vi "PrefDialog.vi"(8 "error in (no error)":errorcluster, 11 "SpecAnPlugins.lvlib":refnum<class "SpecAnBase.lvclass">) -> (0 "error out":errorcluster, 2 "Change Occured?":bool, 3 "SpecAnPlugins.lvlib":refnum<class "SpecAnBase.lvclass">)   [LabVIEW 2018, in "SpecAnPlugins.lvlib" / "SpecAnBase.lvclass"]
doc: "This VI opens up the modal preference dialog window and allows a user to configure the dialog based on a new configuration or the existing configuration that was loaded"
uses:
  SpecAnBase.lvclass
  C:/Program Files (x86)/National Instruments/LabVIEW 2018/user.lib/NIST/BaseClasses/BasePlugin_class/BasePlugin.lvclass
  <userlib>/NIST/BaseClasses/BasePlugin_class/BasePlugin.lvclass/BasePlugin.ctl
  <userlib>/NIST/BaseClasses/BasePlugin_class/Accessors/Read PluginIniFilePath.vi
  <userlib>/NIST/BaseClasses/BasePlugin_class/Accessors/Write PluginIniFilePath.vi
  <vilib>/Utility/config.llb/NI_LVConfig.lvlib
panel:
  in  "btnSave As":bool
  in  "btnSave":bool
  in  "Tab Control":T1(tab)
  in  "Acquisition":T2
  in  "Frequency":T3
  in  "Level":T4
  in  "SweepCoupling":T5
  in  "Trace":T6(array[cluster])
  in  "Trigger":T7
  in  "btnCancel":bool
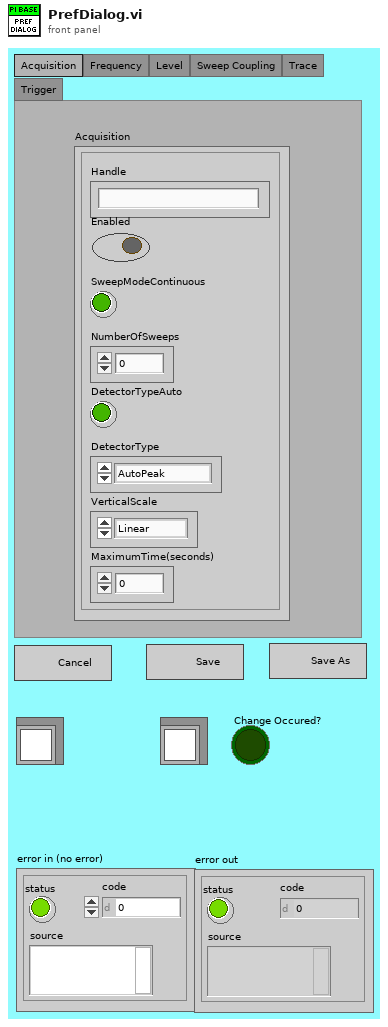
[diagram p1: front panel]
types:
  T1 = enum32{"Acquisition", "Frequency", "Level", "Sweep Coupling", "Trace", "Trigger"}
  T2 = cluster{"Handle":string, "Connected":bool, "Enabled":bool, "SweepModeContinuous":bool, "NumberOfSweeps":i32, "DetectorTypeAuto":bool, "DetectorType":enum16{"AutoPeak", "Average", "MaximumPeak", "MinimumPeak", "Sample", "RMS"}, "VerticalScale":enum16{"Linear", "Logarithmic"}, "MaximumTime(seconds)":dbl}
  T3 = cluster{"FrequencyStart":dbl, "FrequencyStop":dbl, "FrequencyOffset":dbl}
  T4 = cluster{"InputImpedance":dbl, "AttenuationAuto":bool, "AmplitudeUnits":enum16{"dBm", "dBmV", "dBuV", "Volt", "Watt"}, "ReferenceLevel":dbl, "Attenuation":dbl, "ReferenceLevelOffset":dbl}
  T5 = cluster{"ResolutionBandwidth":dbl, "ResolutionBandwidthAuto":bool, "SweepTime":dbl, "VideoBandwidth":dbl, "VideoBandwidthAuto":bool, "SweepTimeAuto":bool}
  T6 = cluster{"TraceName":string, "TraceSize":i32, "TraceType":enum16{"Clear Write", "Maximum Hold", "Minimum Hold", "Video Average", "View", "Store"}}[]
  T7 = cluster{"TriggerSource":string, "TriggerLevel":dbl, "TriggerSlope":enum16{"Positive", "Negative"}}
  T8 = enum8{"Enabled", "Disabled", "Disabled and Grayed Out"}
  T9 = enum32{"Invalid", "Default", "Floating", "Floating/Auto-Hide", "Modal"}
  T10 = typedef "NI_LVConfig.lvlib/Config Data RefNum.ctl" = refnum<k1>
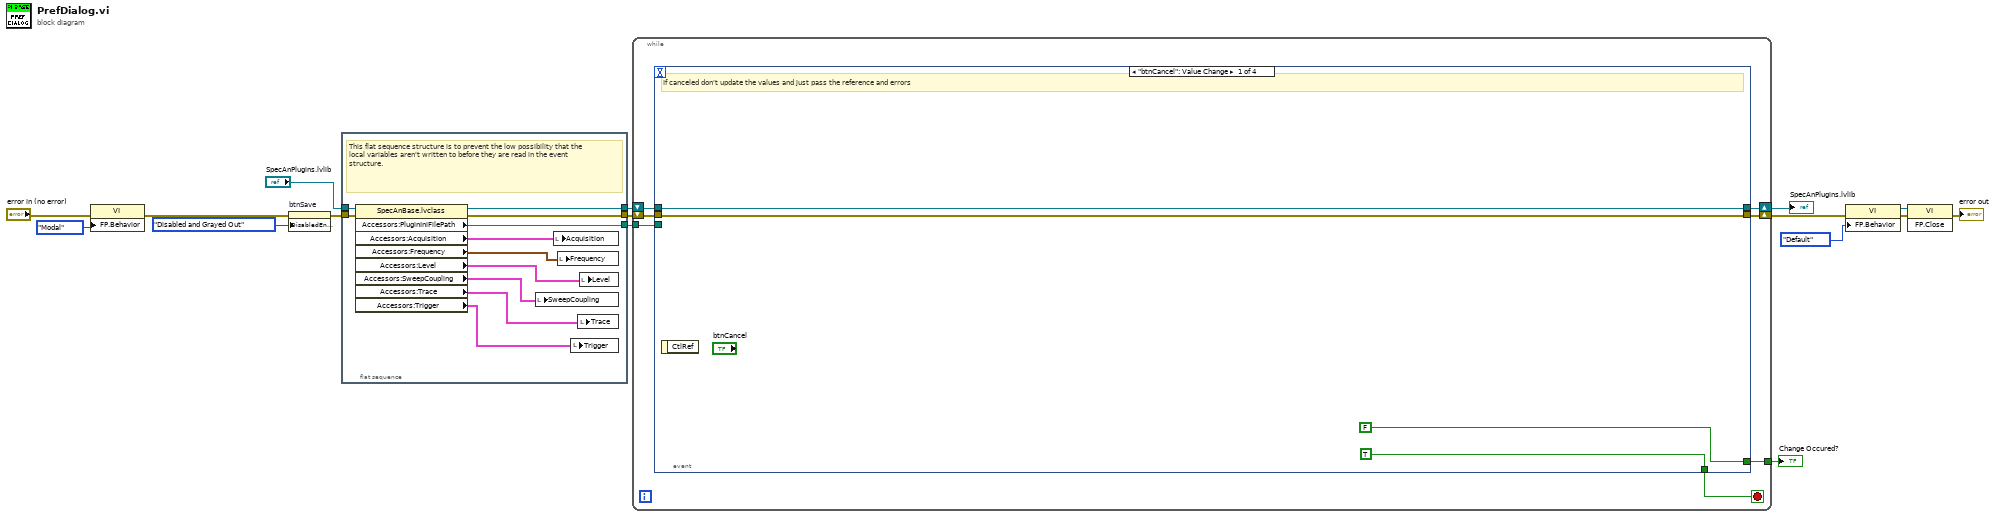
[diagram p0: block diagram]
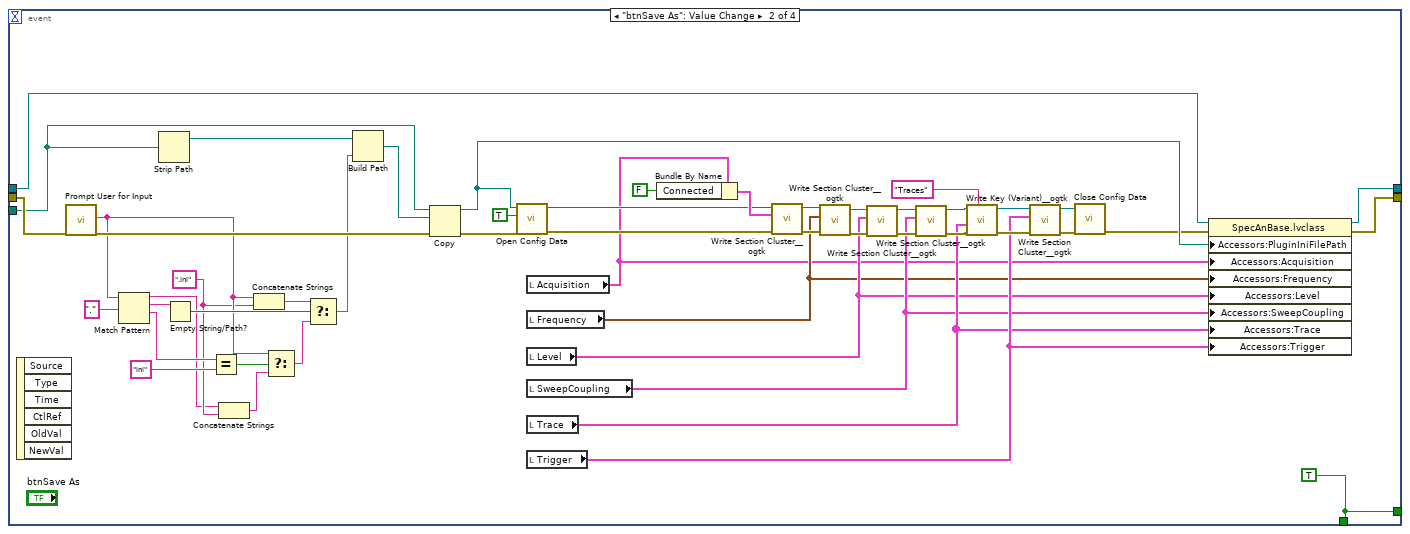
[diagram p2: hidden frame]
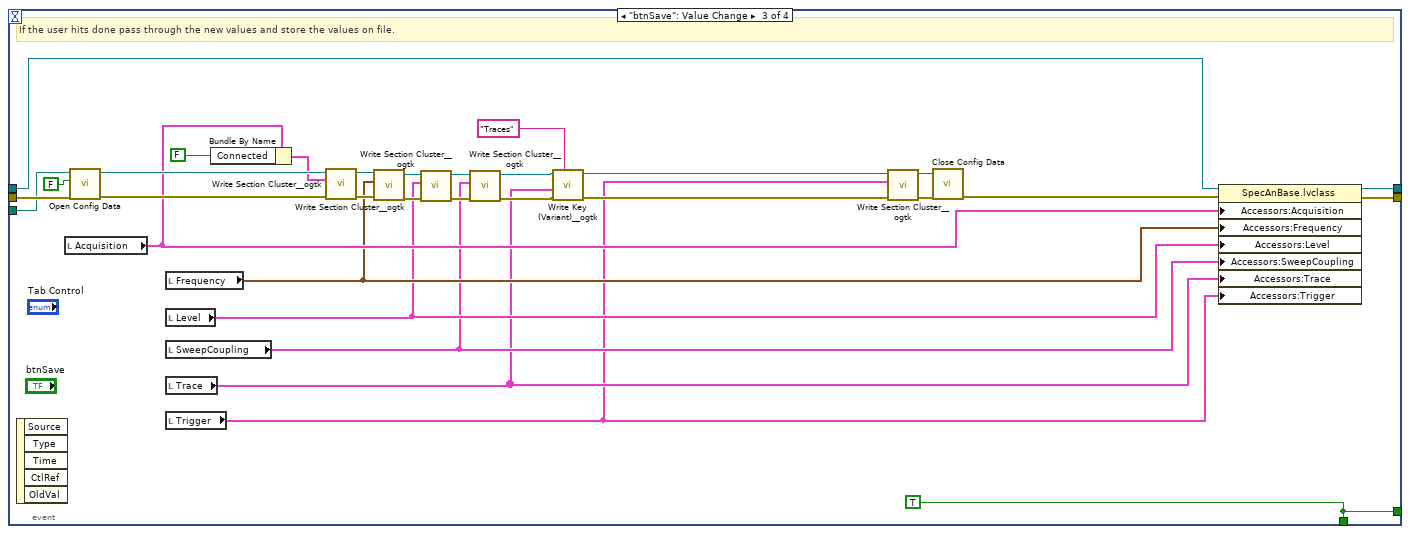
[diagram p3: hidden frame]
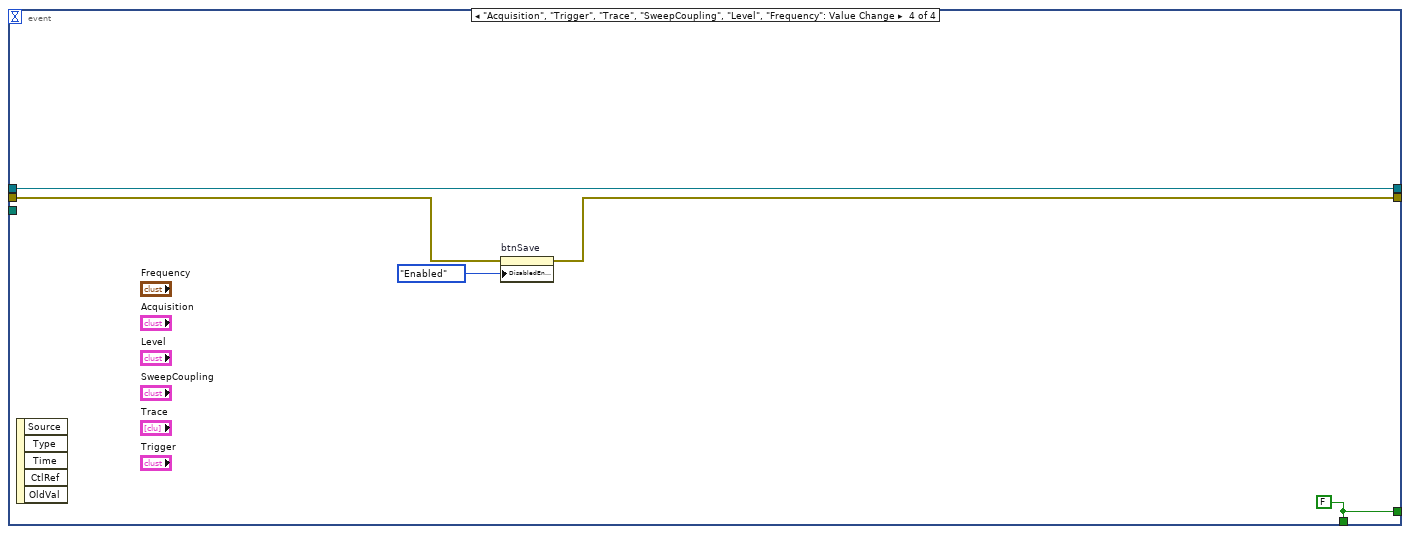
[diagram p4: hidden frame]
diagram:
  n1 = property class="VI"(error in="error in (no error)", "FP.Behavior"=T9."Modal" ("Front Panel Window:Behavior")) -> (error out=w1:errorcluster)  [unwired: 1 in, 1 out]
  n2 = property on="btnSave" class="Bool"(error in=w1, "DisabledEnum"=T8."Disabled and Grayed Out" ("Disabled")) -> (error out=w3:errorcluster)  [unwired: 1 in, 1 out]
  n3 = flat-sequence {
    tunnel: "SpecAnPlugins.lvlib" -> [w27]
    tunnel: w3 -> [w26]
    tunnel: [w25] -> w9
    tunnel: [w24] -> w8
    tunnel: [w23] -> w7
    frame #0 {
      # "This flat sequence structure is to prevent the low possibility that the local variables aren't written to before they are read in the event structure."
      n4 = property class="SpecAnBase.lvclass"(reference=w27, error in=w26) -> (reference out=w24:refnum<class "SpecAnBase.lvclass">, error out=w25:errorcluster, "Accessors:PluginIniFilePath"=w23:path, "Accessors:Acquisition"=w22:T2, "Accessors:Frequency"=w21:T3, "Accessors:Level"=w20:T4, "Accessors:SweepCoupling"=w19:T5, "Accessors:Trace"=w18:T6, "Accessors:Trigger"=w17:T7)
      n5 = local write "SweepCoupling"(w19) -> ()
      n6 = local write "Acquisition"(w22) -> ()
      n7 = local write "Frequency"(w21) -> ()
      n8 = local write "Trigger"(w17) -> ()
      n9 = local write "Trace"(w18) -> ()
      n10 = local write "Level"(w20) -> ()
    }
  }
  n11 = while {
    tunnel: w7 -> [w32]
    shift-right: [w30] -> w5
    shift-left: w9 -> [w34]
    shift-right: [w31] -> w6
    shift-left: w8 -> [w33]
    tunnel: [w28] -> w4
    stop <- w29 stop-if-true
    n12 = event shown="[0] \"btnCancel\": Value Change" {
      selector: _ -> [_ _ _ _]
      dyn-events: _ -> [_ _ _ _]
      timeout: _ -> [_ _ _ _]
      tunnel: w34 -> [w37 w84 w110 w122]
      tunnel: w33 -> [w38 w47 w118 w123]
      tunnel: w32 -> [_ w82 w102 _]
      tunnel: [w38 w86 w117 w123] -> w31
      tunnel: [w37 w85 w116 w121] -> w30
      tunnel: [TRUE w87 w94 w119] -> w29
      tunnel: [FALSE w87 w94 w119] -> w28
      event "btnCancel": Value Change {
        # "If canceled don't update the values and just pass the reference and errors"
        n13 = event-data() -> ()  [unwired: 1 in, 1 out]
      }
      event "btnSave As": Value Change {
        w69 = ".ini" ("string")
        w87 = TRUE
        n14 = event-data() -> ()  [unwired: 1 in, 6 out]
        n15 = call "Prompt User for Input"("error in (no error)"=w84) -> ("File Name"=w75:string, "error out"=w80:errorcluster)  [unwired: 15 in, 2 out]
        n16 = Match Pattern(string=w75, regular expression="." ("string")) -> (before substring=w68:string, match substring=w72:string, after substring=w71:string)  [unwired: 1 in, 1 out]
        n17 = Strip Path(path=w82) -> (stripped path=w83:path)  [unwired: 1 out]
        n18 = Empty String/Path?(string/path=w72) -> (empty?=w79:bool)
        n19 = Equal?(x=w71, y="ini" ("string")) -> (x = y?=w76:bool)
        n20 = Concatenate Strings(w68, w69) -> (w67:string)
        n21 = Concatenate Strings(w75, w69) -> (w78:string)
        n22 = Select(t=w75, s=w76, f=w67) -> (s? t:f=w74:string)
        n23 = Select(t=w78, s=w79, f=w74) -> (s? t:f=w77:string)
        n24 = Build Path(base path=w83, name or relative path=w77) -> (appended path=w81:path)
        n25 = Copy(8:w80, 10:w81, 11:w82) -> (0:w65:errorcluster, 3:w64:path)  [unwired: 2 in, 1 out]
        n26 = call <vilib>:"Open Config Data.vi"("error in (no error)"=w65, "create file if necessary (T)"=TRUE, "configuration file path"=w64) -> ("error out"=w46:errorcluster, "refnum"=w45:T10)  [unwired: 6 in, 1 out]
        n27 = local read "Acquisition"() -> (w39:T2)
        n28 = local read "Frequency"() -> (w40:T3)
        n29 = local read "Level"() -> (w41:T4)
        n30 = local read "SweepCoupling"() -> (w42:T5)
        n31 = local read "Trace"() -> (w43:T6)
        n32 = local read "Trigger"() -> (w44:T7)
        n33 = Bundle By Name(cluster=w39, "Connected"=FALSE) -> (w51:T2)
        n34 = call <userlib>:"Write Section Cluster__ogtk.vi"("error in (no error)"=w46, "Section Formatted Cluster"=w51, "refnum"=w45) -> ("error out"=w63:errorcluster, "dup refnum"=w62:T10)  [unwired: 7 in]
        n35 = call <userlib>:"Write Section Cluster__ogtk.vi"("error in (no error)"=w63, "Section Formatted Cluster"=w40, "refnum"=w62) -> ("error out"=w61:errorcluster, "dup refnum"=w60:T10)  [unwired: 7 in]
        n36 = call <userlib>:"Write Section Cluster__ogtk.vi"("error in (no error)"=w61, "Section Formatted Cluster"=w41, "refnum"=w60) -> ("error out"=w59:errorcluster, "dup refnum"=w58:T10)  [unwired: 7 in]
        n37 = call <userlib>:"Write Section Cluster__ogtk.vi"("error in (no error)"=w59, "Section Formatted Cluster"=w42, "refnum"=w58) -> ("error out"=w55:errorcluster, "dup refnum"=w54:T10)  [unwired: 7 in]
        n38 = call <userlib>:"Write Key (Variant)__ogtk.vi"("section"="Traces", "error in (no error)"=w55, "key-value"=w43, "refnum"=w54) -> ("error out"=w53:errorcluster, "refnum out"=w52:T10)  [unwired: 6 in]
        n39 = call <userlib>:"Write Section Cluster__ogtk.vi"("error in (no error)"=w53, "Section Formatted Cluster"=w44, "refnum"=w52) -> ("error out"=w57:errorcluster, "dup refnum"=w56:T10)  [unwired: 7 in]
        n40 = call <vilib>:"Close Config Data.vi"("error in (no error)"=w57, "refnum"=w56) -> ("error out"=w48:errorcluster)  [unwired: 8 in, 1 out]
        n41 = property class="SpecAnBase.lvclass"(reference=w47, error in=w48, "Accessors:PluginIniFilePath"=w64, "Accessors:Acquisition"=w39, "Accessors:Frequency"=w40, "Accessors:Level"=w41, "Accessors:SweepCoupling"=w42, "Accessors:Trace"=w43, "Accessors:Trigger"=w44) -> (reference out=w86:refnum<class "SpecAnBase.lvclass">, error out=w85:errorcluster)
      }
      event "btnSave": Value Change {
        w94 = TRUE
        # "If the user hits done pass through the new values and store the values on file."
        n42 = event-data() -> ()  [unwired: 1 in, 5 out]
        n43 = local read "Acquisition"() -> (w93:T2)
        n44 = call <vilib>:"Open Config Data.vi"("error in (no error)"=w110, "create file if necessary (T)"=FALSE, "configuration file path"=w102) -> ("error out"=w113:errorcluster, "refnum"=w112:T10)  [unwired: 6 in, 1 out]
        n45 = local read "Frequency"() -> (w92:T3)
        n46 = local read "Level"() -> (w91:T4)
        n47 = local read "SweepCoupling"() -> (w90:T5)
        n48 = local read "Trace"() -> (w89:T6)
        n49 = local read "Trigger"() -> (w88:T7)
        n50 = Bundle By Name(cluster=w93, "Connected"=FALSE) -> (w95:T2)
        n51 = call <userlib>:"Write Section Cluster__ogtk.vi"("error in (no error)"=w113, "Section Formatted Cluster"=w95, "refnum"=w112) -> ("error out"=w115:errorcluster, "dup refnum"=w114:T10)  [unwired: 7 in]
        n52 = call <userlib>:"Write Section Cluster__ogtk.vi"("error in (no error)"=w115, "Section Formatted Cluster"=w92, "refnum"=w114) -> ("error out"=w108:errorcluster, "dup refnum"=w107:T10)  [unwired: 7 in]
        n53 = call <userlib>:"Write Section Cluster__ogtk.vi"("error in (no error)"=w108, "Section Formatted Cluster"=w91, "refnum"=w107) -> ("error out"=w106:errorcluster, "dup refnum"=w105:T10)  [unwired: 7 in]
        n54 = call <userlib>:"Write Section Cluster__ogtk.vi"("error in (no error)"=w106, "Section Formatted Cluster"=w90, "refnum"=w105) -> ("error out"=w101:errorcluster, "dup refnum"=w100:T10)  [unwired: 7 in]
        n55 = call <userlib>:"Write Key (Variant)__ogtk.vi"("section"="Traces", "error in (no error)"=w101, "key-value"=w89, "refnum"=w100) -> ("error out"=w98:errorcluster, "refnum out"=w97:T10)  [unwired: 6 in]
        n56 = call <userlib>:"Write Section Cluster__ogtk.vi"("error in (no error)"=w98, "Section Formatted Cluster"=w88, "refnum"=w97) -> ("error out"=w104:errorcluster, "dup refnum"=w103:T10)  [unwired: 7 in]
        n57 = call <vilib>:"Close Config Data.vi"("error in (no error)"=w104, "refnum"=w103) -> ("error out"=w109:errorcluster)  [unwired: 8 in, 1 out]
        n58 = property class="SpecAnBase.lvclass"(reference=w118, error in=w109, "Accessors:Acquisition"=w93, "Accessors:Frequency"=w92, "Accessors:Level"=w91, "Accessors:SweepCoupling"=w90, "Accessors:Trace"=w89, "Accessors:Trigger"=w88) -> (reference out=w117:refnum<class "SpecAnBase.lvclass">, error out=w116:errorcluster)
      }
      event "Acquisition", "Trigger", "Trace", "SweepCoupling", "Level", "Frequency": Value Change {
        w119 = FALSE
        n59 = event-data() -> ()  [unwired: 1 in, 5 out]
        n60 = property on="btnSave" class="Bool"(error in=w122, "DisabledEnum"=T8."Enabled" ("Disabled")) -> (error out=w121:errorcluster)  [unwired: 1 in, 1 out]
      }
    }
  }
  "SpecAnPlugins.lvlib" <- w6
  "Change Occured?" <- w4
  n61 = property class="VI"(error in=w5, "FP.Behavior"=T9."Default" ("Front Panel Window:Behavior")) -> (reference out=w11:refnum<vi>, error out=w14:errorcluster)  [unwired: 1 in]
  n62 = invoke class="VI" method="FP.Close"(reference=w11, error in=w14) -> (error out=→"error out":errorcluster)  [unwired: 1 in, 2 out]
